vi "advent_3.vi"() -> ()   [LabVIEW 2021]
uses:
  <vilib>/Utility/file.llb/Read Delimited Spreadsheet (string).vi
panel:
  out "Array 4":i32[][](array[numeric])
  out "Array 3":i32[][](array[numeric])
  out "subarray":i32[](array[numeric])
  out "Array 2":i32[][](array[numeric])
  out "Array":i32[][](array[numeric])
  out "nujmber of 1's 2":i32
  out "size(s) 3":i32
  out "nujmber of 1's":i32
  out "size(s) 2":i32
  out "x*y":u32
  out "epsilon n":u32
  out "epsilon":bool[](array[boolean])
  out "gamma n":u32
  out "gamma":bool[](array[boolean])
  out "Nmber 0":i32[](array[numeric])
  out "number of 1's":i32[](array[numeric])
  out "size(s)":i32
  # "900"
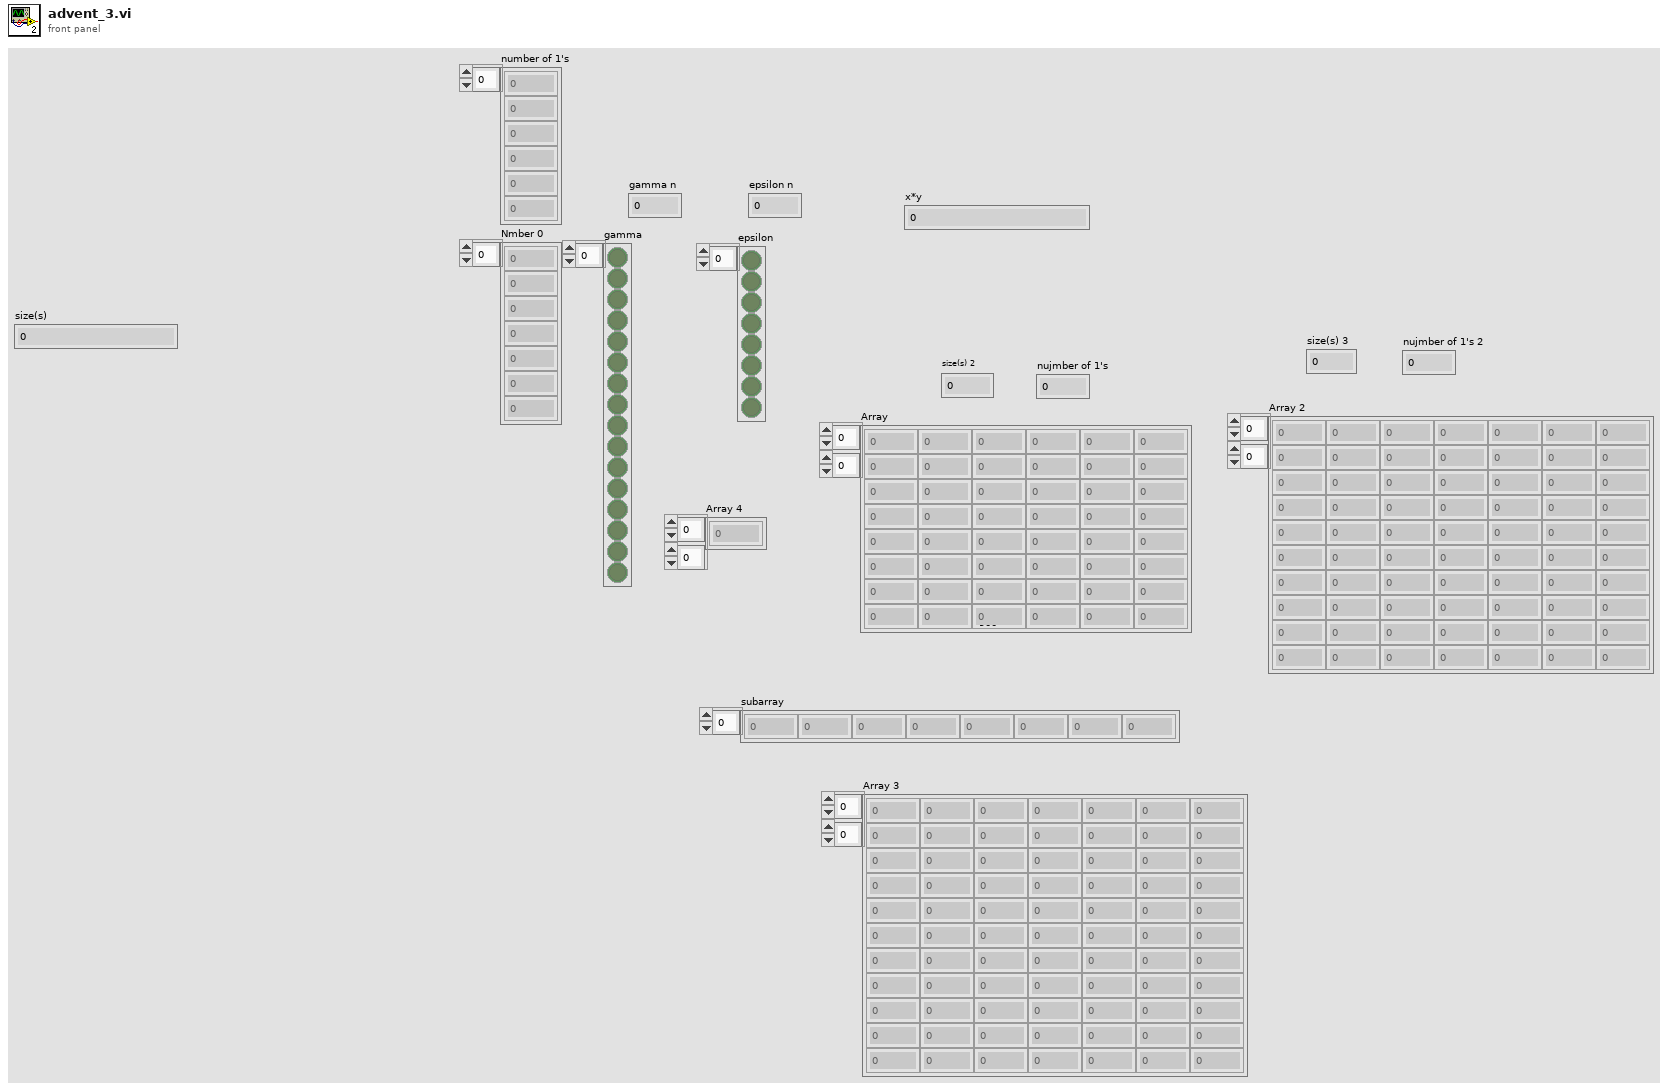
[diagram p1: front panel]
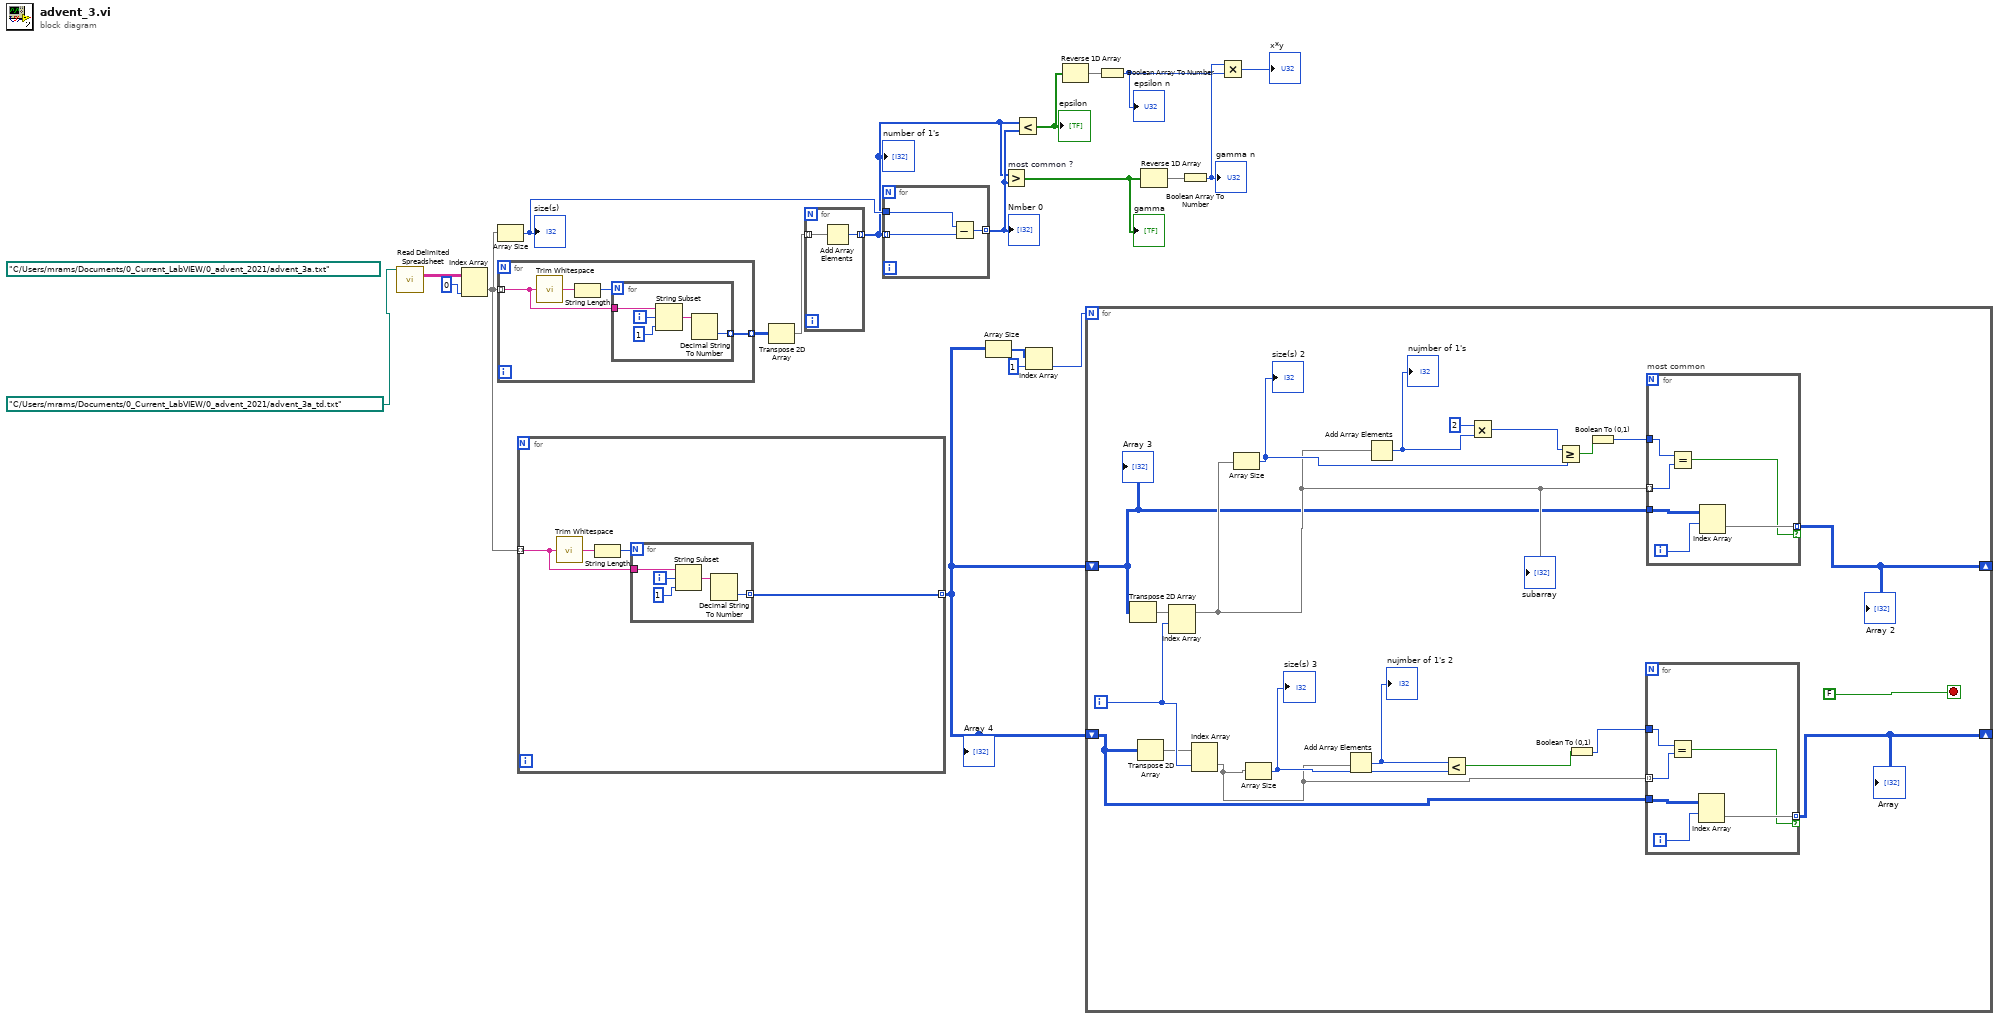
[diagram p0: block diagram]
diagram:
  (unwired) path "C:/Users/mrams/Documents/0_Current_LabVIEW/0_advent_2021/advent_3a.txt" ("file path (dialog if empty)")
  n1 = call-poly <vilib>:"Read Delimited Spreadsheet.vi"("file path (dialog if empty)"=path "C:/Users/mrams/Documents/0_Current_LabVIEW/0_advent_2021/advent_3a_td.txt") -> ("all rows"=w19:string[][])  [unwired: 9 in, 5 out]
  n2 = Index Array(array=w19, index (col)=0 ("disabled index (col)")) -> (element=w6:string[])  [unwired: 1 in]
  n3 = Array Size(array=w6) -> (size(s)=w16:i32)
  "size(s)" <- w16
  n4 = for {
    tunnel: w6 -> [w24] mode=indexing
    tunnel: [w21] -> w18 mode=indexing
    n5 = call <vilib>:"Trim Whitespace.vi"("string"=w24) -> ("trimmed string"=w22:string)  [unwired: 1 in]
    n6 = String Length(string=w22) -> (length=w23:i32)
    n7 = for {
      N: w23 -> [_]
      tunnel: w24 -> [w29]
      tunnel: [w25] -> w21 mode=indexing
      i -> [w28]
      n8 = String Subset(string=w29, offset (0)=w28, length (rest)=1 ("length (rest)")) -> (substring=w27:string)
      n9 = Decimal String To Number(string=w27) -> (number=w25:i32)  [unwired: 2 in, 1 out]
    }
  }
  n10 = for {
    tunnel: w6 -> [w33] mode=indexing
    tunnel: [w30] -> w5 mode=indexing
    n11 = call <vilib>:"Trim Whitespace.vi"("string"=w33) -> ("trimmed string"=w31:string)  [unwired: 1 in]
    n12 = String Length(string=w31) -> (length=w32:i32)
    n13 = for {
      N: w32 -> [_]
      tunnel: w33 -> [w38]
      tunnel: [w34] -> w30 mode=indexing
      i -> [w37]
      n14 = String Subset(string=w38, offset (0)=w37, length (rest)=1 ("length (rest)")) -> (substring=w36:string)
      n15 = Decimal String To Number(string=w36) -> (number=w34:i32)  [unwired: 2 in, 1 out]
    }
  }
  "Array 4" <- w5
  n16 = Transpose 2D Array(2D array=w18) -> (transposed array=w17:i32[][])
  n17 = for {
    tunnel: w17 -> [w40] mode=indexing
    tunnel: [w39] -> w13 mode=indexing
    n18 = Add Array Elements(numeric array=w40) -> (sum=w39:i32)
  }
  "number of 1's" <- w13
  n19 = for {
    tunnel: w13 -> [w42] mode=indexing
    tunnel: w16 -> [w43]
    tunnel: [w41] -> w14 mode=indexing
    n20 = Subtract(x=w43, y=w42) -> (x-y=w41:i32)
  }
  "Nmber 0" <- w14
  n21 = Array Size(array=w5) -> (size(s)=w4:i32[])
  n22 = Greater? "most common ?"(x=w13, y=w14) -> (0:w15:bool[])
  "gamma" <- w15
  n23 = Less?(x=w13, y=w14) -> (x < y?=w12:bool[])
  "epsilon" <- w12
  n24 = Index Array(array=w4, index=1) -> (element=w2:i32)
  n25 = Reverse 1D Array(array=w12) -> (reversed array=w8:bool[])
  n26 = for {
    N: w2 -> [_]
    shift-right: [w61] -> _
    shift-left: w5 -> [w59]
    shift-right: [w51] -> _
    shift-left: w5 -> [w52]
    i -> [w56]
    stop <- FALSE stop-if-true
    n27 = Transpose 2D Array(2D array=w59) -> (transposed array=w48:i32[][])
    n28 = Transpose 2D Array(2D array=w52) -> (transposed array=w47:i32[][])
    n29 = Index Array(array=w48, index (row)=w56) -> (element=w60:i32[])  [unwired: 1 in]
    "subarray" <- w60
    n30 = Index Array(array=w47, index (row)=w56) -> (element=w49:i32[])  [unwired: 1 in]
    n31 = Array Size(array=w60) -> (size(s)=w63:i32)
    "size(s) 2" <- w63
    n32 = Array Size(array=w49) -> (size(s)=w53:i32)
    "size(s) 3" <- w53
    n33 = Add Array Elements(numeric array=w49) -> (sum=w54:i32)
    "nujmber of 1's 2" <- w54
    n34 = Add Array Elements(numeric array=w60) -> (sum=w46:i32)
    "nujmber of 1's" <- w46
    n35 = Less?(x=w54, y=w53) -> (x < y?=w55:bool)
    n36 = Multiply(x=2, y=w46) -> (x*y=w44:i32)
    n37 = Greater Or Equal?(x=w44, y=w63) -> (x >= y?=w62:bool)
    n38 = Boolean To (0,1)(Boolean=w55) -> (0, 1=w50:i16)
    n39 = Boolean To (0,1)(Boolean=w62) -> (0, 1=w57:i16)
    n40 = for {
      tunnel: w49 -> [w65] mode=indexing
      tunnel: w50 -> [w66]
      tunnel: w52 -> [w69]
      tunnel: [w67] -> w51 mode=indexing if=w64
      i -> [w68]
      n41 = Equal?(x=w66, y=w65) -> (x = y?=w64:bool)
      n42 = Index Array(array=w69, index (row)=w68) -> (element=w67:i32[])  [unwired: 1 in]
    }
    "Array" <- w51
    n43 = for "most common" {
      tunnel: w60 -> [w71] mode=indexing
      tunnel: w57 -> [w72]
      tunnel: w59 -> [w75]
      tunnel: [w73] -> w61 mode=indexing if=w70
      i -> [w74]
      n44 = Equal?(x=w72, y=w71) -> (x = y?=w70:bool)
      n45 = Index Array(array=w75, index (row)=w74) -> (element=w73:i32[])  [unwired: 1 in]
    }
    "Array 2" <- w61
    "Array 3" <- w59
  }
  n46 = Boolean Array To Number(Boolean array=w8) -> (number=w10:u32)
  "epsilon n" <- w10
  n47 = Reverse 1D Array(array=w15) -> (reversed array=w7:bool[])
  n48 = Boolean Array To Number(Boolean array=w7) -> (number=w11:u32)
  "gamma n" <- w11
  n49 = Multiply(x=w11, y=w10) -> (x*y=→"x*y":u32)
